vi "Test Server Restart.vi"() -> ()   [LabVIEW 2020, in "VectoScratch.lvlib"]
uses:
  VectoScratch.lvlib
  Vecto/LocalEventCollector/Event.ctl
  lv-volatus/Volatus/Event Level.ctl
  Vecto/Event Level.ctl
  f55d3f37-42f4-4a3f-8c10-89cbbd344fc8.vi
  Vecto/LocalEventCollector/LocalEventCollector.lvclass
  C:/dev/lv20CE/relink/lv-vecto/Vecto/EventLogHandler/EventLogHandler.lvclass
  Vecto/TCPMessaging/TCPMessaging.lvclass
  Vecto/SequenceCountService/SequenceCountService.lvclass
  Vecto/EventLoggingService/EventLoggingService.lvclass
  Vecto/Vecto.lvlib
  lv-volatus/Volatus/Volatus.lvlib
panel:
  out "error out":errorcluster
  in  "Stop":bool
  in  "Restart":bool
  out "Events":T1[](array[typedef])
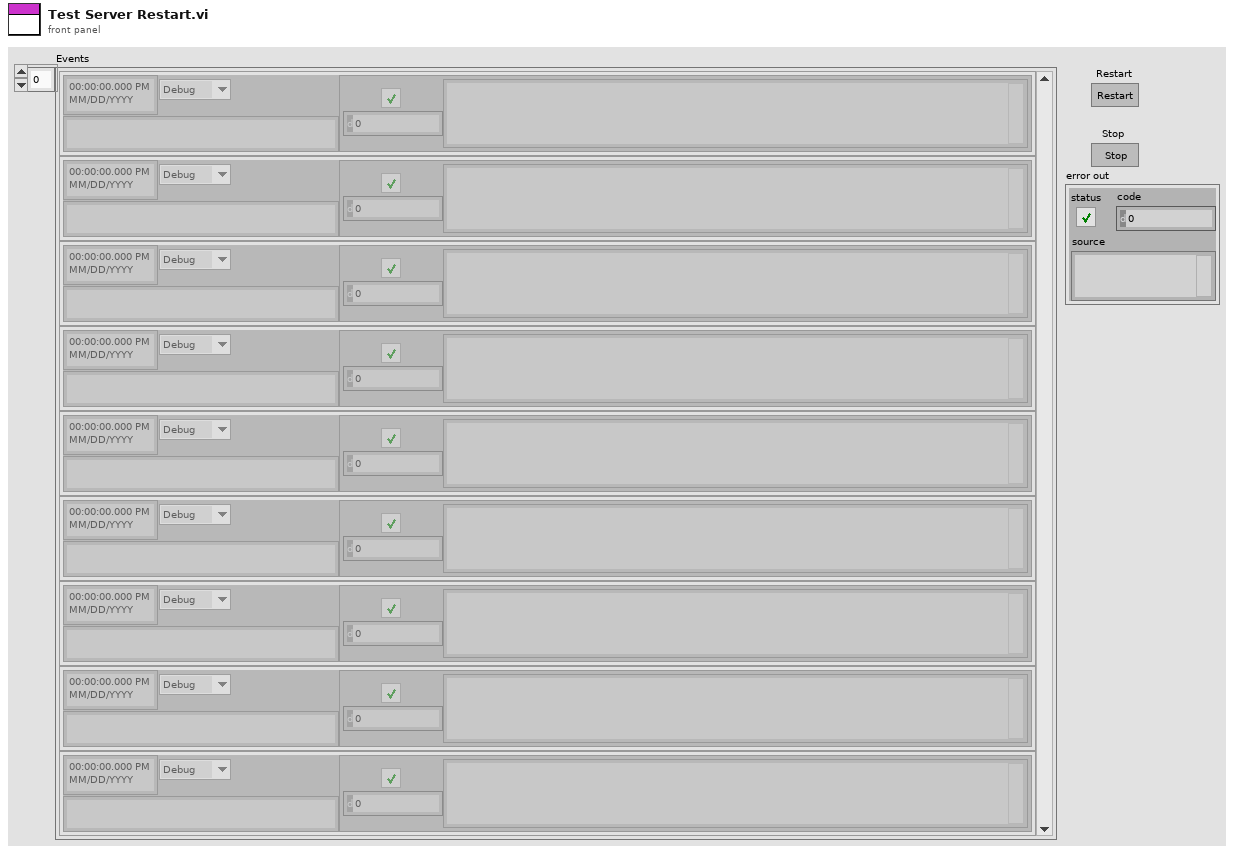
[diagram p1: front panel]
types:
  T1 = typedef "Vecto.lvlib/LocalEventCollector.lvclass/Event.ctl" = cluster{"Time Stamp":timestamp, "Event Level":T2, "Message":string, "Error":errorcluster}
  T2 = typedef "Volatus.lvlib/Event Level.ctl" = enum16{"Debug", "Info", "Warning", "Error"}
  T3 = typedef "Vecto.lvlib/Event Level.ctl" = enum16{"Debug", "Info", "Warning", "Error"}
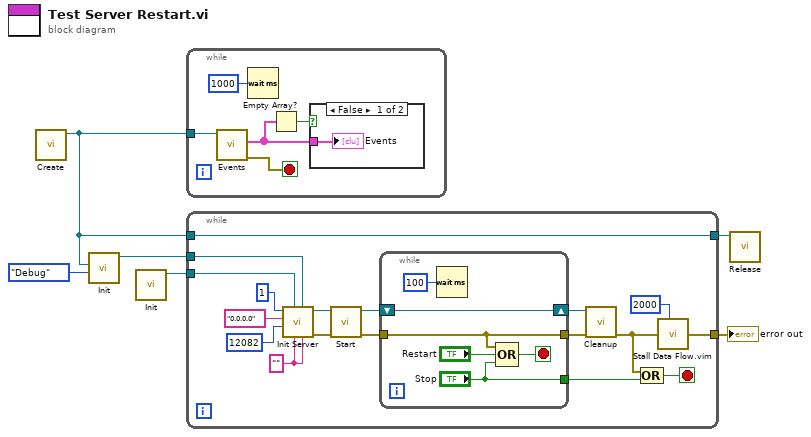
[diagram p0: block diagram]
diagram:
  n1 = call "Create.vi"() -> ("LocalEventCollector out"=w4:refnum<class "LocalEventCollector.lvclass">)  [unwired: 10 in, 1 out]
  n2 = call "Init.vi"("Minimum Event Level"=Event_Level."Debug", "EventLogger"=w4) -> ("EventLoggingService out"=w5:refnum<class "EventLoggingService.lvclass">)  [unwired: 8 in, 1 out]
  n3 = call "Init.vi"() -> ("SequenceCountService out"=w6:refnum<class "SequenceCountService.lvclass">)  [unwired: 10 in, 1 out]
  n4 = while {
    tunnel: w4 -> [w11]
    stop <- w10 stop-if-true
    n5 = call "Events.vi"("LocalEventCollector in"=w11) -> ("error out"=w10:errorcluster, "Events"=w8:T1[])  [unwired: 8 in, 1 out]
    n6 = Wait (ms)(milliseconds to wait=u32 1000) -> ()  [unwired: 1 out]
    n7 = Empty Array?(array=w8) -> (empty?=w7:bool)
    n8 = case shown="False" w7 {
      tunnel: w8 -> [w12 _]
      frame False {
        "Events" <- w12
      }
      frame True {
      }
    }
  }
  n9 = while {
    tunnel: w6 -> [w29]
    tunnel: w5 -> [w28]
    tunnel: [w14] -> w2
    tunnel: w4 -> [w15]
    tunnel: [w15] -> w3
    stop <- w16 stop-if-true
    w25 = "" ("Local Config Version")
    n10 = call "Init Server.vi"("Local Config Hash"=w25, "EventLogger"=w28, "Local Config Version"=w25, "SequenceCountService"=w29, "Bind Port"=u16 12082, "Bind Address"="0.0.0.0", "Node ID"=u32 1) -> ("error out"=w24:errorcluster, "TCPMessaging out"=w23:refnum<class "TCPMessaging.lvclass">)  [unwired: 3 in]
    n11 = call "Start.vi"("error in (no error)"=w24, "TCPMessaging in"=w23) -> ("error out"=w22:errorcluster, "TCPMessaging out"=w21:refnum<class "TCPMessaging.lvclass">)  [unwired: 8 in]
    n12 = while {
      tunnel: w22 -> [w33]
      shift-right: [w35] -> w19
      shift-left: w21 -> [w35]
      tunnel: [w33] -> w20
      tunnel: ["Stop"] -> w17
      stop <- w34 stop-if-true
      n13 = Wait (ms)(milliseconds to wait=u32 100) -> ()  [unwired: 1 out]
      n14 = Compound Arithmetic op=OR(w33, "Restart", "Stop") -> (w34:bool)
    }
    n15 = call "Cleanup.vi"("error in (no error)"=w20, "TCPMessaging in"=w19) -> ("error out"=w18:errorcluster)  [unwired: 9 in]
    n16 = Compound Arithmetic op=OR(w18, w17) -> (w16:bool)
    n17 = call "Stall Data Flow.vim"("value in"=w18, "milliseconds to wait"=u32 2000) -> ("value out"=w14:errorcluster)  [unwired: 1 out]
  }
  "error out" <- w2
  n18 = call "Release.vi"("LocalEventCollector in"=w3) -> ()  [unwired: 10 in, 1 out]
